vi "Acquire_OSCILL_SubVI_3CH.vi"(6 "Vertical Scale[mV] CH3":dbl=5.0, 8 "error in (no error)":errorcluster, 9 "Vertical Scale[mV] CH1":dbl=5.0, 10 "N_acquisition":i32, 11 "VISA resource name":refnum<visa-resource-name>) -> (0 "error out":errorcluster, 1 "Time":dbl[](array[numeric]), 2 "CH2_averaged":dbl[](array[numeric]), 3 "CH1_averaged":dbl[](array[numeric]), 4 "CH3_averaged":dbl[](array[numeric]), 5 "VISA resource name out":refnum<visa-resource-name>)   [LabVIEW 2017]
uses:
  Agilent 2000 3000 X-Series/Agilent 2000 3000 X-Series.lvlib
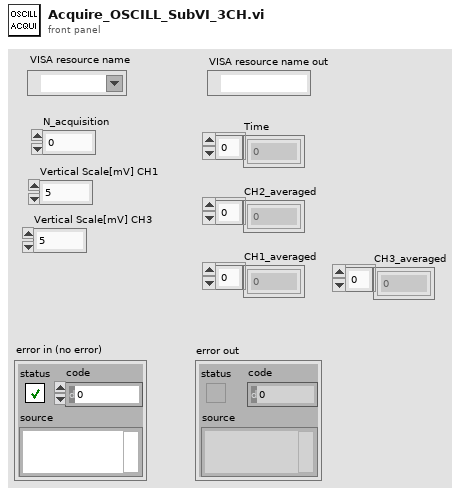
[diagram p1: front panel]
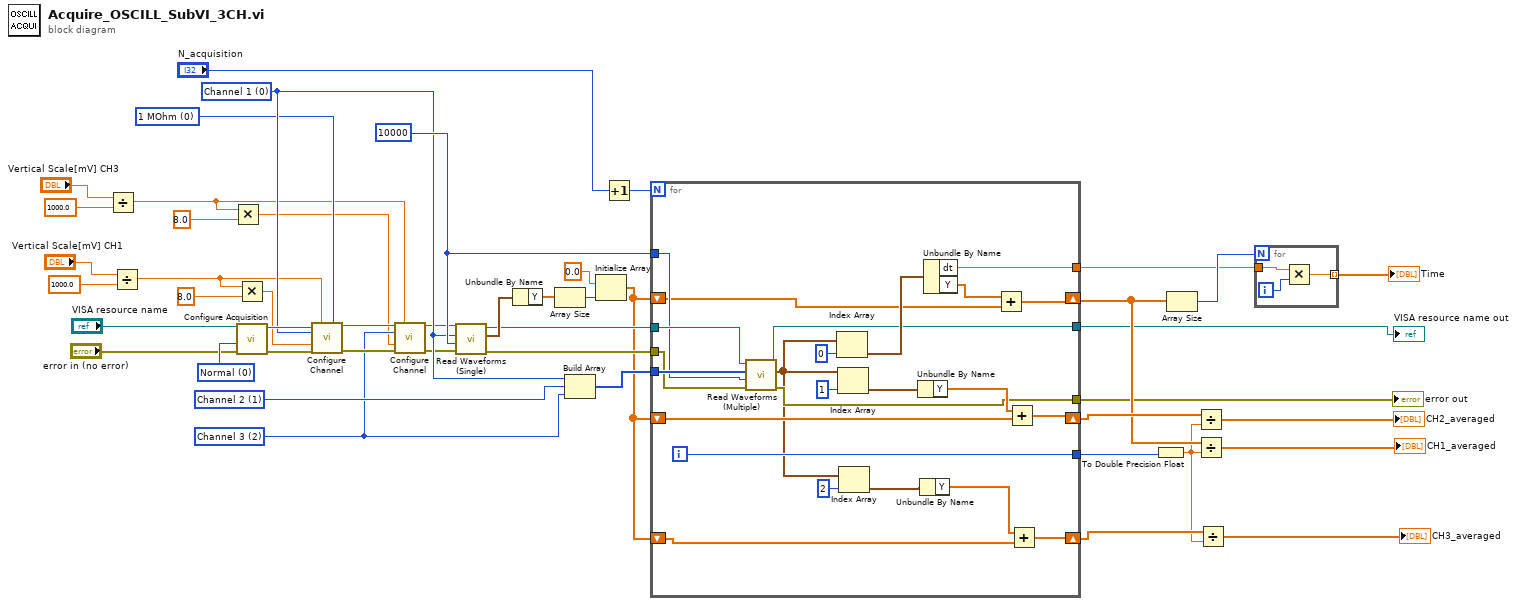
[diagram p0: block diagram]
diagram:
  w10 = 2 items=["Channel 1"=0, "Channel 2"=1, "Channel 3"=2, "Channel 4"=3, "Digital Bus Low"=9, "Digital Bus High"=10] ("Source Channel (0: Channel 1)")
  w19 = 0 items=["1 MOhm", "50 Ohm"] ("Impedance (0: 1 MOhm)")
  w29 = 1 items=["Channel 1"=0, "Channel 2"=1, "Channel 3"=2, "Channel 4"=3, "Digital Bus Low"=9, "Digital Bus High"=10] ("Source Channel (0: Channel 1)")
  w30 = 0 items=["Channel 1"=0, "Channel 2"=1, "Channel 3"=2, "Channel 4"=3, "Digital Bus Low"=9, "Digital Bus High"=10] ("Source Channel (0: Channel 1)")
  w46 = 0 items=["Normal", "Average", "High Resolution", "Peak"] ("Acquisition Type (0: Normal)")
  w47 = u32 10000 ("y")
  n1 = Divide(x="Vertical Scale[mV] CH3", y=1000.0) -> (x/y=w3:dbl)
  n2 = Divide(x="Vertical Scale[mV] CH1", y=1000.0) -> (x/y=w9:dbl)
  n3 = Multiply(x=w3, y=8.0) -> (x*y=w4:dbl)
  n4 = Multiply(x=w9, y=8.0) -> (x*y=w8:dbl)
  n5 = call "Configure Acquisition.vi"("error in (no error)"="error in (no error)", "Acquisition Type (0: Normal)"=w46, "VISA resource name"="VISA resource name") -> ("error out"=w38:errorcluster, "VISA resource name out"=w39:refnum<visa-resource-name>)  [unwired: 7 in]
  n6 = call "Configure Channel.vi"("VISA resource name"=w39, "Vertical Scale (5.0 V)"=w9, "Impedance (0: 1 MOhm)"=w19, "Channel Name (0: Channel 1)"=w30, "Vertical Range (40.0 V)"=w8, "error in (no error)"=w38) -> ("VISA resource name out"=w12:refnum<visa-resource-name>, "error out"=w14:errorcluster)  [unwired: 5 in, 3 out]
  n7 = call "Configure Channel.vi"("VISA resource name"=w12, "Vertical Scale (5.0 V)"=w3, "Channel Name (0: Channel 1)"=w10, "Vertical Range (40.0 V)"=w4, "error in (no error)"=w14) -> ("VISA resource name out"=w11:refnum<visa-resource-name>, "error out"=w13:errorcluster)  [unwired: 6 in, 3 out]
  n8 = call "Read Waveforms (Single).vi"("error in (no error)"=w13, "Timeout (10000 ms)"=w47, "Source Channel (0: Channel 1)"=w30, "VISA resource name"=w11) -> ("error out"=w34:errorcluster, "Waveform Data"=w43:waveform(dbl), "VISA resource name out"=w33:refnum<visa-resource-name>)  [unwired: 1 in, 4 out]
  n9 = Unbundle By Name(w43) -> ("Y"=w44:dbl[])
  n10 = Array Size(array=w44) -> (size(s)=w45:i32)
  n11 = Build Array(w30, w29, w10) -> (w28:i32[])
  n12 = Initialize Array(0.0 ("element"), w45) -> (w18:dbl[])
  n13 = Increment(x="N_acquisition") -> (x+1=w41:i32)
  n14 = for {
    N: w41 -> [_]
    tunnel: w47 -> [w68]
    shift-right: [w61] -> w22
    shift-left: w18 -> [w59]
    tunnel: [w71] -> w24
    shift-right: [w57] -> w23
    shift-left: w18 -> [w56]
    tunnel: w34 -> [w67]
    tunnel: w33 -> [w70]
    tunnel: w28 -> [w69]
    tunnel: [w62] -> w26
    tunnel: [w55] -> w21
    tunnel: [w54] -> w20
    shift-right: [w49] -> w17
    shift-left: w18 -> [w48]
    i -> [w71]
    n15 = call "Read Waveforms (Multiple).vi"("error in (no error)"=w67, "Timeout (10000 ms)"=w68, "Channels"=w69, "VISA resource name"=w70) -> ("error out"=w54:errorcluster, "Waveform Data"=w52:waveform(dbl)[], "VISA resource name out"=w55:refnum<visa-resource-name>)  [unwired: 5 out]
    n16 = Index Array(array=w52, index=0) -> (element=w63:waveform(dbl))
    n17 = Index Array(array=w52, index=1) -> (element=w64:waveform(dbl))
    n18 = Index Array(array=w52, index=2) -> (element=w51:waveform(dbl))
    n19 = Unbundle By Name(w64) -> ("Y"=w58:dbl[])
    n20 = Unbundle By Name(w51) -> ("Y"=w50:dbl[])
    n21 = Unbundle By Name(w63) -> ("dt"=w62:dbl, "Y"=w60:dbl[])
    n22 = Add(x=w60, y=w59) -> (x+y=w61:dbl[])
    n23 = Add(x=w58, y=w56) -> (x+y=w57:dbl[])
    n24 = Add(x=w50, y=w48) -> (x+y=w49:dbl[])
  }
  "error out" <- w20
  "VISA resource name out" <- w21
  n25 = To Double Precision Float(number=w24) -> (double precision float=w16:dbl)
  n26 = Array Size(array=w22) -> (size(s)=w27:i32)
  n27 = Divide(x=w23, y=w16) -> (x/y=→"CH2_averaged":dbl[])
  n28 = Divide(x=w22, y=w16) -> (x/y=→"CH1_averaged":dbl[])
  n29 = Divide(x=w17, y=w16) -> (x/y=→"CH3_averaged":dbl[])
  n30 = for {
    N: w27 -> [_]
    tunnel: w26 -> [w73]
    tunnel: [w74] -> w25 mode=indexing
    i -> [w72]
    n31 = Multiply(x=w73, y=w72) -> (x*y=w74:dbl)
  }
  "Time" <- w25
